vi "LVClass_SlopesPostProcessList GetProcessorListName.vi"(0 "SlopesPostProcessorList in":refnum<class "SlopesPostProcessorList.lvclass">, 11 "error in (no error)":errorcluster) -> (4 "SlopesPostProcessorList out":refnum<class "SlopesPostProcessorList.lvclass">, 6 "name":string[](array[string]), 15 "error out":errorcluster)   [LabVIEW 2020, in "SlopesPostProcessorList.lvclass"]
doc: "Get names of the the SlopesPostProcessors contained into the\nSlopesPostProcessorList.\n\n--------------------------------------------------------------------------------\n\n<B>SlopesPostProcessorListIn </B> : SlopesPostProcessorList object.\n<B>SlopesPostProcessorListOut </B> : SlopesPostProcessorList object.\n<B>listname </B> : List of processors names.\n<B>ErrorIn </B> : Error\n<B>ErrorOut </B> : Error\n\n--------------------------------------------------------------------------------"
uses:
  SlopesPostProcessorList.lvclass
  SlopesPostProcessorList.lvclass/SlopesPostProcessorList.ctl
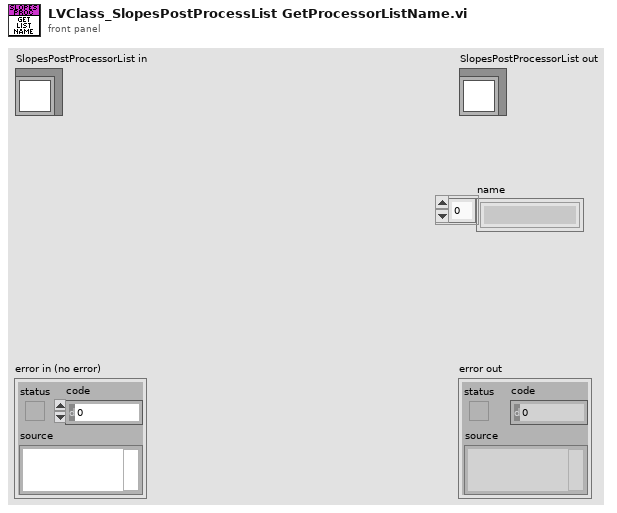
[diagram p1: front panel]
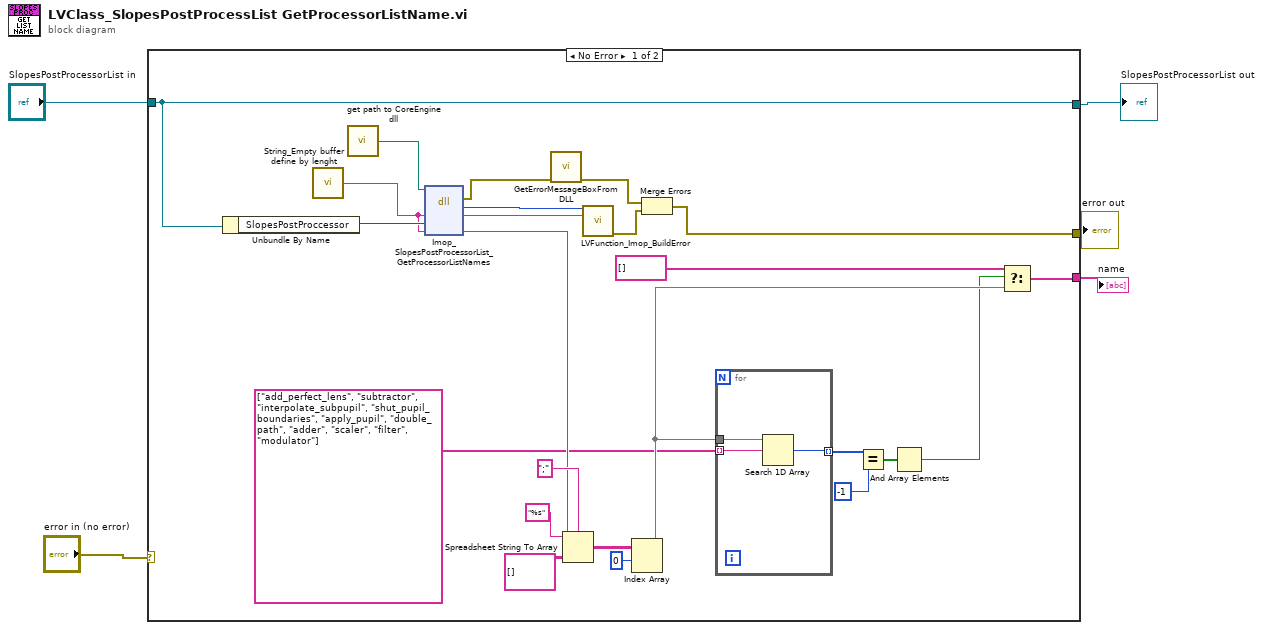
[diagram p0: block diagram]
diagram:
  n1 = case shown="No Error" "error in (no error)" {
    selector: "error in (no error)" -> [_ w33]
    tunnel: "SlopesPostProcessorList in" -> [w25 w34]
    tunnel: [w25 w34] -> w3
    tunnel: [w16 w33] -> w2
    tunnel: [w12 _] -> w1
    frame No Error {
      n2 = Unbundle By Name(w25) -> ("SlopesPostProccessor"=w24:i32)
      n3 = call "String_Empty buffer define by lenght.vi"() -> ("Empty buffer"=w14:string)  [unwired: 1 in]
      n4 = call "get path to CoreEngine dll.vi"() -> ("path to c_interface_vc100.dll"=w27:path)  [unwired: 12 in, 3 out]
      n5 = dll-call lib="D:/soft/HASO_v3/SVN_trunk/ImOpCoreEngine4_LV2011/DLLs/c_interface_vc100.dll" fn="Imop_SlopesPostProcessorList_GetProcessorListNames"(path in=w27, "message"=w14, "objet"=w24, "name"=w14) -> (error out=w26:errorcluster, "return type"=w28:i32, "message"=w29:string, "name"=w15:string)  [unwired: 3 in, 1 out]
      n6 = call "GetErrorMessageBoxFromDLL.vi"("error IN"=w26) -> ("error OUT"=w18:errorcluster)  [unwired: 10 in]
      n7 = Spreadsheet String To Array(delimiter (Tab)=";", format string="%s", spreadsheet string=w15, array type (2D Dbl)=string[][] []) -> (array=w20:string[][])
      n8 = call "LVFunction_Imop_BuildError.vi"("code"=w28, "String to Prepend to source (\"\")"=w29) -> ("error out"=w17:errorcluster)  [unwired: 13 in]
      n9 = Index Array(array=w20, index (row)=0) -> (element=w11:string[])  [unwired: 1 in]
      n10 = Merge Errors(w18, w17) -> (w16:errorcluster)
      n11 = for {
        tunnel: w11 -> [w32]
        tunnel: string[] ["add_perfect_lens", "subtractor", "interpolate_subpupil", "shut_pupil_boundaries", "apply_pupil", "double_path", "adder", "scaler", "filter", "modulator"] -> [w31] mode=indexing
        tunnel: [w30] -> w9 mode=indexing
        n12 = Search 1D Array(1D array=w32, element=w31) -> (index of element=w30:i32)  [unwired: 1 in]
      }
      n13 = Equal?(x=w9, y=-1 ("index of element")) -> (x = y?=w7:bool[])
      n14 = And Array Elements(Boolean array=w7) -> (logical AND=w6:bool)
      n15 = Select(t=string[] [], s=w6, f=w11) -> (s? t:f=w12:string[])
    }
    frame Error {
    }
  }
  "error out" <- w2
  "SlopesPostProcessorList out" <- w3
  "name" <- w1
